vi "main.vi"() -> ()   [LabVIEW 2022 SP3]
uses:
  <vilib>/ptbypt/NI_PtbyPt.lvlib
panel:
  out "Sequenza tasti premuti":string
  out "Waveform Chart":dbl(graph)
  out "error out":errorcluster
  in  "error in (no error)":errorcluster
  in  "Boolean 12":bool
  in  "Boolean 11":bool
  in  "Boolean 10":bool
  in  "Boolean 9":bool
  in  "Boolean 8":bool
  in  "Boolean 7":bool
  in  "Boolean 6":bool
  in  "Boolean 5":bool
  in  "Boolean 4":bool
  in  "Boolean 3":bool
  in  "Boolean 2":bool
  in  "Boolean":bool
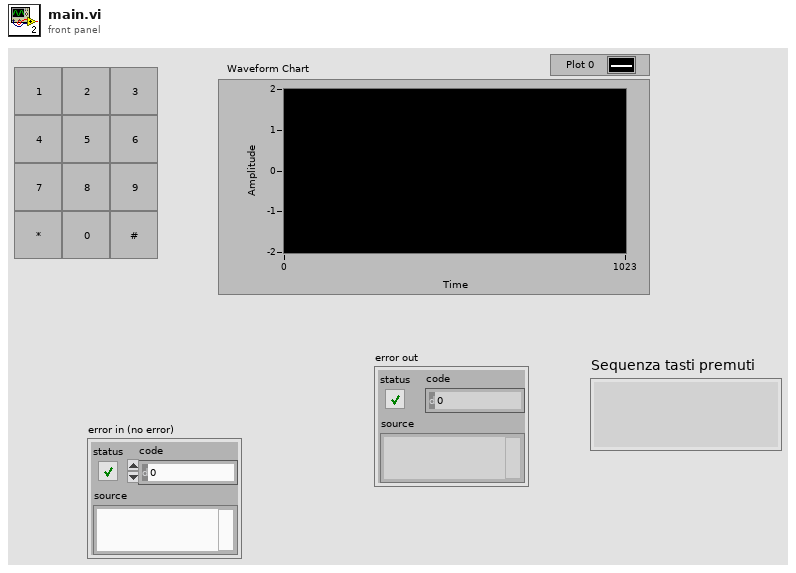
[diagram p1: front panel]
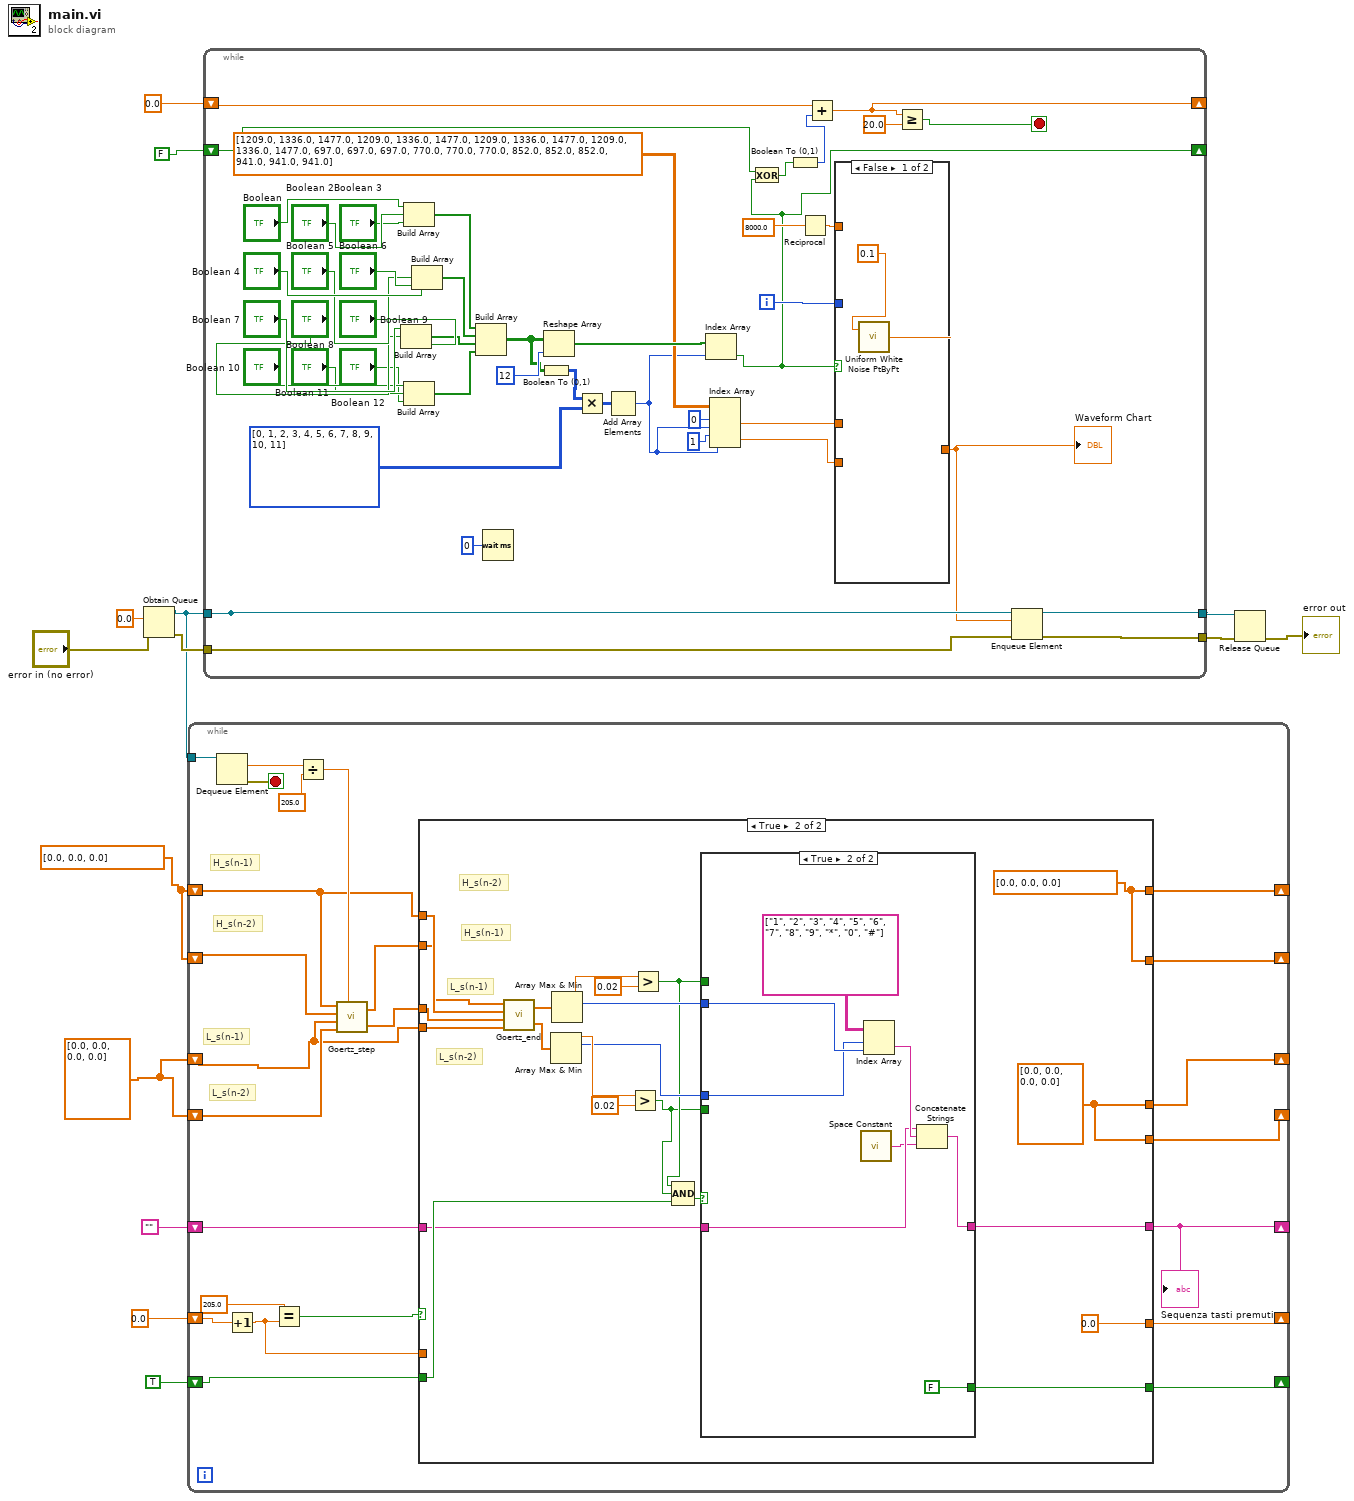
[diagram p0: block diagram]
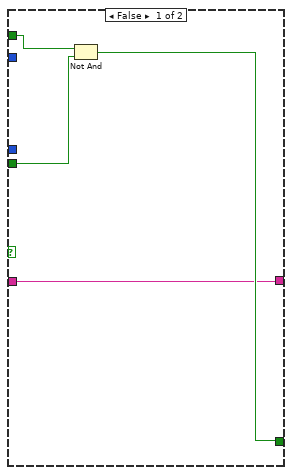
[diagram p3: hidden frame]
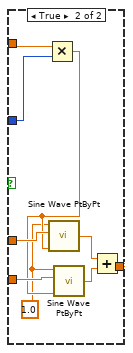
[diagram p4: hidden frame]
diagram:
  w2 = dbl[] [0.0, 0.0, 0.0, 0.0]
  w1 = dbl[] [0.0, 0.0, 0.0]
  n1 = Obtain Queue(element data type=0.0, error in (no error)="error in (no error)") -> (queue out=w6:refnum<queue>, error out=w12:errorcluster)  [unwired: 3 in, 1 out]
  n2 = while {
    tunnel: w6 -> [w38]
    shift-right: [w21] -> _
    shift-left: w1 -> [w32]
    shift-right: [w18] -> _
    shift-left: w2 -> [w34]
    shift-right: [w17] -> _
    shift-left: "" -> [w24]
    shift-right: [w15] -> _
    shift-left: 0.0 -> [w29]
    shift-right: [w16] -> _
    shift-left: TRUE -> [w25]
    shift-right: [w19] -> _
    shift-left: w2 -> [w23]
    shift-right: [w20] -> _
    shift-left: w1 -> [w22]
    stop <- w37 stop-if-true
    # "L_s(n-2)"
    # "L_s(n-1)"
    # "H_s(n-2)"
    # "H_s(n-1)"
    n3 = Dequeue Element(queue=w38) -> (element=w36:dbl, error out=w37:errorcluster)  [unwired: 2 in, 2 out]
    n4 = Increment(x=w29) -> (x+1=w26:dbl)
    n5 = Equal?(x=205.0, y=w26) -> (x = y?=w27:bool)
    n6 = Divide(x=w36, y=205.0) -> (x/y=w33:dbl)
    n7 = call "Goertz_step.vi"("H_s(n-1)"=w32, "H_s(n-2)"=w22, "L_s(n-1)"=w23, "L_s(n-2)"=w34, "x(n)"=w33) -> ("H_s(n)"=w31:dbl[], "L_s(n)"=w30:dbl[])
    n8 = case shown="True" w27 {
      tunnel: w32 -> [w44 w65]
      tunnel: w31 -> [w45 w64]
      tunnel: w30 -> [w43 w67]
      tunnel: w23 -> [w42 w66]
      tunnel: w26 -> [w40 _]
      tunnel: w25 -> [w39 w53]
      tunnel: w24 -> [w41 w51]
      tunnel: [w45 w50] -> w21
      tunnel: [w44 w50] -> w20
      tunnel: [w43 w49] -> w19
      tunnel: [w42 w49] -> w18
      tunnel: [w41 w48] -> w17
      tunnel: [w39 w47] -> w16
      tunnel: [w40 0.0] -> w15
      frame False {
      }
      frame True {
        w49 = dbl[] [0.0, 0.0, 0.0, 0.0]
        w50 = dbl[] [0.0, 0.0, 0.0]
        # "L_s(n-2)"
        # "L_s(n-1)"
        # "H_s(n-1)"
        # "H_s(n-2)"
        n9 = call "Goertz_end.vi"("L_s(n-2)"=w66, "L_s(n-1)"=w67, "H_s(n-2)"=w65, "H_s(n-1)"=w64) -> ("L_mag"=w62:dbl[], "H_mag"=w63:dbl[])
        n10 = Array Max & Min(array=w62) -> (max value=w58:dbl, max index (indices)=w57:i32)  [unwired: 2 out]
        n11 = Array Max & Min(array=w63) -> (max value=w61:dbl, max index (indices)=w56:i32)  [unwired: 2 out]
        n12 = Greater?(x=w58, y=0.02) -> (0:w54:bool)
        n13 = Greater?(x=w61, y=0.02) -> (0:w55:bool)
        n14 = Compound Arithmetic op=AND(w55, w54, w53) -> (w52:bool)
        n15 = case shown="True" w52 {
          tunnel: w55 -> [w71 _]
          tunnel: w54 -> [w70 _]
          tunnel: w57 -> [_ w73]
          tunnel: w56 -> [_ w74]
          tunnel: w51 -> [w68 w77]
          tunnel: [w69 FALSE] -> w47
          tunnel: [w68 w75] -> w48
          frame False {
            n16 = Not And(1:w70, 2:w71) -> (0:w69:bool)
          }
          frame True {
            n17 = call <vilib>:"Space Constant.vi"() -> ("String"=w72:string)
            n18 = Index Array(array=string[][] [["1", "2", "3"], ["4", "5", "6"], ["7", "8", "9"], ["*", "0", "#"]], index (row)=w73, index (col)=w74) -> (element=w78:string)
            n19 = Concatenate Strings(w77, w78, w72) -> (w75:string)
          }
        }
      }
    }
    "Sequenza tasti premuti" <- w17
  }
  n20 = while {
    tunnel: [w93] -> _
    tunnel: w6 -> [w93]
    tunnel: w12 -> [w92]
    tunnel: [w91] -> w11
    tunnel: [w90] -> w10
    shift-right: [w84] -> _
    shift-left: 0.0 -> [w89]
    shift-right: [w82] -> _
    shift-left: FALSE -> [w83]
    i -> [w96]
    stop <- w85 stop-if-true
    n21 = Build Array("Boolean 7", "Boolean 8", "Boolean 9") -> (w110:bool[])
    n22 = Build Array("Boolean", "Boolean 2", "Boolean 3") -> (w112:bool[])
    n23 = Build Array("Boolean 10", "Boolean 11", "Boolean 12") -> (w109:bool[])
    n24 = Build Array("Boolean 4", "Boolean 5", "Boolean 6") -> (w111:bool[])
    n25 = Build Array(w112, w111, w110, w109) -> (w107:bool[][])
    n26 = Wait (ms)(milliseconds to wait=u32 0) -> ()  [unwired: 1 out]
    n27 = Boolean To (0,1)(Boolean=w107) -> (0, 1=w106:i16[][])
    n28 = Reshape Array(w107, 12 ("dimension size")) -> (w103:bool[])
    n29 = Multiply(x=w106, y=i16[][] [[0, 1, 2], [3, 4, 5], [6, 7, 8], [9, 10, 11]]) -> (x*y=w104:i16[][])
    n30 = Add Array Elements(numeric array=w104) -> (sum=w99:i16)
    n31 = Index Array(array=w103, index=w99) -> (element=w82:bool)
    n32 = Index Array(array=dbl[][] [[1209.0, 1336.0, 1477.0, 1209.0, 1336.0, 1477.0, 1209.0, 1336.0, 1477.0, 1209.0, 1336.0, 1477.0], [697.0, 697.0, 697.0, 770.0, 770.0, 770.0, 852.0, 852.0, 852.0, 941.0, 941.0, 941.0]], index (row) #1=0 ("disabled index (row)"), index (col) #1=w99, index (row) #2=1 ("index (row)"), index (col) #2=w99) -> (element #1=w95:dbl, element #2=w94:dbl)
    n33 = Exclusive Or(1:w82, 2:w83) -> (0:w88:bool)
    n34 = Boolean To (0,1)(Boolean=w88) -> (0, 1=w87:i16)
    n35 = Reciprocal(x=8000.0) -> (1/x=w97:dbl)
    n36 = Add(x=w89, y=w87) -> (x+y=w84:dbl)
    n37 = case shown="False" w82 {
      tunnel: w97 -> [_ w135]
      tunnel: w96 -> [_ w134]
      tunnel: w95 -> [_ w133]
      tunnel: w94 -> [_ w132]
      tunnel: [w126 w127] -> w81
      frame False {
        n38 = call <vilib>:"Uniform White Noise PtByPt.vi"("amplitude"=0.1) -> ("uniform white noise"=w126:dbl)  [unwired: 2 in]
      }
      frame True {
        w130 = 1.0
        n39 = Multiply(x=w135, y=w134) -> (x*y=w131:dbl)
        n40 = call <vilib>:"Sine Wave PtByPt.vi"("time"=w131, "frequency"=w133, "amplitude"=w130) -> ("sine wave"=w129:dbl)  [unwired: 1 in]
        n41 = call <vilib>:"Sine Wave PtByPt.vi"("time"=w131, "frequency"=w132, "amplitude"=w130) -> ("sine wave"=w128:dbl)  [unwired: 1 in]
        n42 = Add(x=w129, y=w128) -> (x+y=w127:dbl)
      }
    }
    "Waveform Chart" <- w81
    n43 = Greater Or Equal?(x=w84, y=20.0) -> (x >= y?=w85:bool)
    n44 = Enqueue Element(queue=w93, element=w81, error in (no error)=w92) -> (queue out=w91:refnum<queue>, error out=w90:errorcluster)  [unwired: 1 in, 1 out]
  }
  n45 = Release Queue(queue=w11, error in (no error)=w10) -> (error out=→"error out":errorcluster)  [unwired: 1 in, 2 out]
